vi "Chain3.vi"(7 "Name (\"\" to Use UUID)":string="CSM-Module") -> ()   [LabVIEW 2017, in "CSM-Testcase.lvlib"]
doc: "Creates a template for a CSM module without a user interface.\n\n> [!NOTE] CSM Name Rules\n> - The CSM module name must be unique to avoid entering the \"Critical Error\" state.\n> - If the input is \"\", a UUID will be used as the module name. This module will operate in independent mode and will not be listed in the module list.\n> - If the input ends with '#', the module will run in work mode. Modules with the same name will share the same message queue. External messages will be handled by the idle module.\n\n> [!NOTE] CSM Initialization State\n> - The default value is \"Macro: Initialize\", consistent with the JKISM state machine.\n> - This state is typically not modified and is provided to facilitate external programmatic changes to the initialization state.\n\n\n-- <b>Controls</b> --\n- <b>Name (\"\" to Use UUID)</b>: CSM Module Name\n- <b>Init State(\"Macro: Initialize\")</b>: Initialization State, default is \"Macro: Initialize\""
uses:
  CSM-Testcase.lvlib
  src/user.lib/_NEVSTOP/Communicable State Machine(CSM)/AdvanceAPI/CSM - Revert Arguments-Safe String.vi
  src/user.lib/_NEVSTOP/Communicable State Machine(CSM)/AdvanceAPI/CSM - Make String Arguments Safe.vi
  src/user.lib/_NEVSTOP/Communicable State Machine(CSM)/AdvanceAPI/CSM - Break Down Multiple States String.vi
  src/user.lib/_NEVSTOP/Communicable State Machine(CSM)/AdvanceAPI/CSM - Keywords.vi
  src/user.lib/_NEVSTOP/Communicable State Machine(CSM)/_Shared/Trim Single-line Text.vi
  src/user.lib/_NEVSTOP/Communicable State Machine(CSM)/_Polymophic/Build No-Reply Asynchronous Message with Arguments.vi
  src/user.lib/_NEVSTOP/Communicable State Machine(CSM)/_Polymophic/Build Asynchronous Message with Arguments.vi
  src/user.lib/_NEVSTOP/Communicable State Machine(CSM)/_Polymophic/Build Interrupt Broadcast Message.vi
  src/user.lib/_NEVSTOP/Communicable State Machine(CSM)/_Polymophic/Build Register Message.vi
  src/user.lib/_NEVSTOP/Communicable State Machine(CSM)/Communicable State Machine.lvlib
  src/user.lib/_NEVSTOP/Communicable State Machine(CSM)/addons/Loop-Support/CSM Loop Support.lvlib
panel:
  out "Error Occurred":errorcluster
  out "State History":string
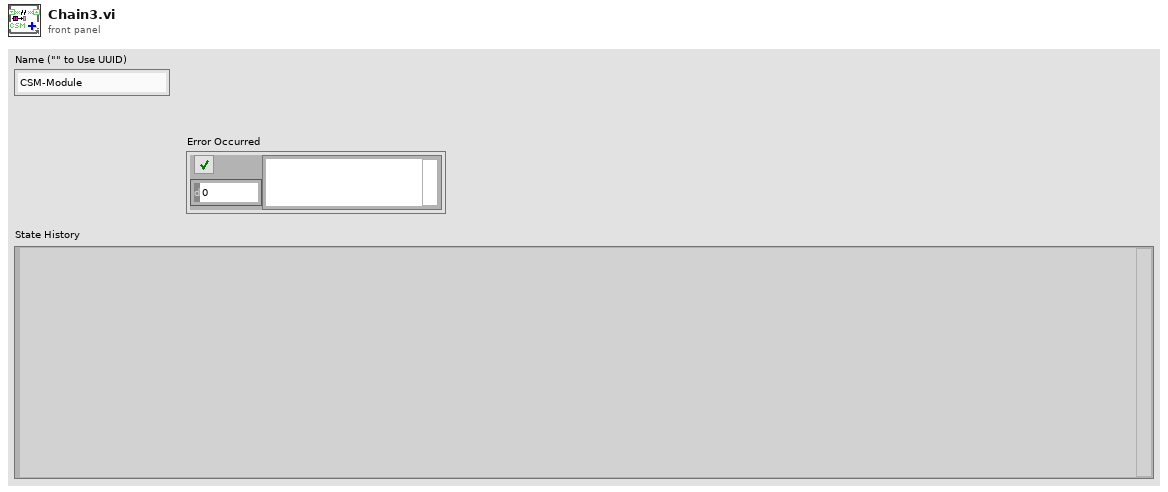
[diagram p1: front panel]
types:
  T1 = cluster{"Arguments":string, "Response":string, "error":errorcluster}
  T2 = enum32{"Invalid", "Standard", "Closed", "Hidden", "Minimized", "Maximized"}
  T3 = enum32{"invalid app kind", "Development System", "Run Time System", "Student Edition", "Embedded LabVIEW", "Evaluation", "Custom"}
  T4 = typedef "Communicable State Machine.lvlib/_CSM_Response Source Message.ctl" = cluster{"‘State":string, "’Arguments":string, "’Error":errorcluster}
  T5 = cluster{"Current VI Reference":refnum<vi>, "Close Panel on Exit?":bool}
  T6 = cluster{"Core":cluster{"Current VI Reference":refnum<vi>, "Close Panel on Exit?":bool}, "Your Boolean data":bool, "Your string data":string, "Counter":u32, "CSM Loop Counter":i32}
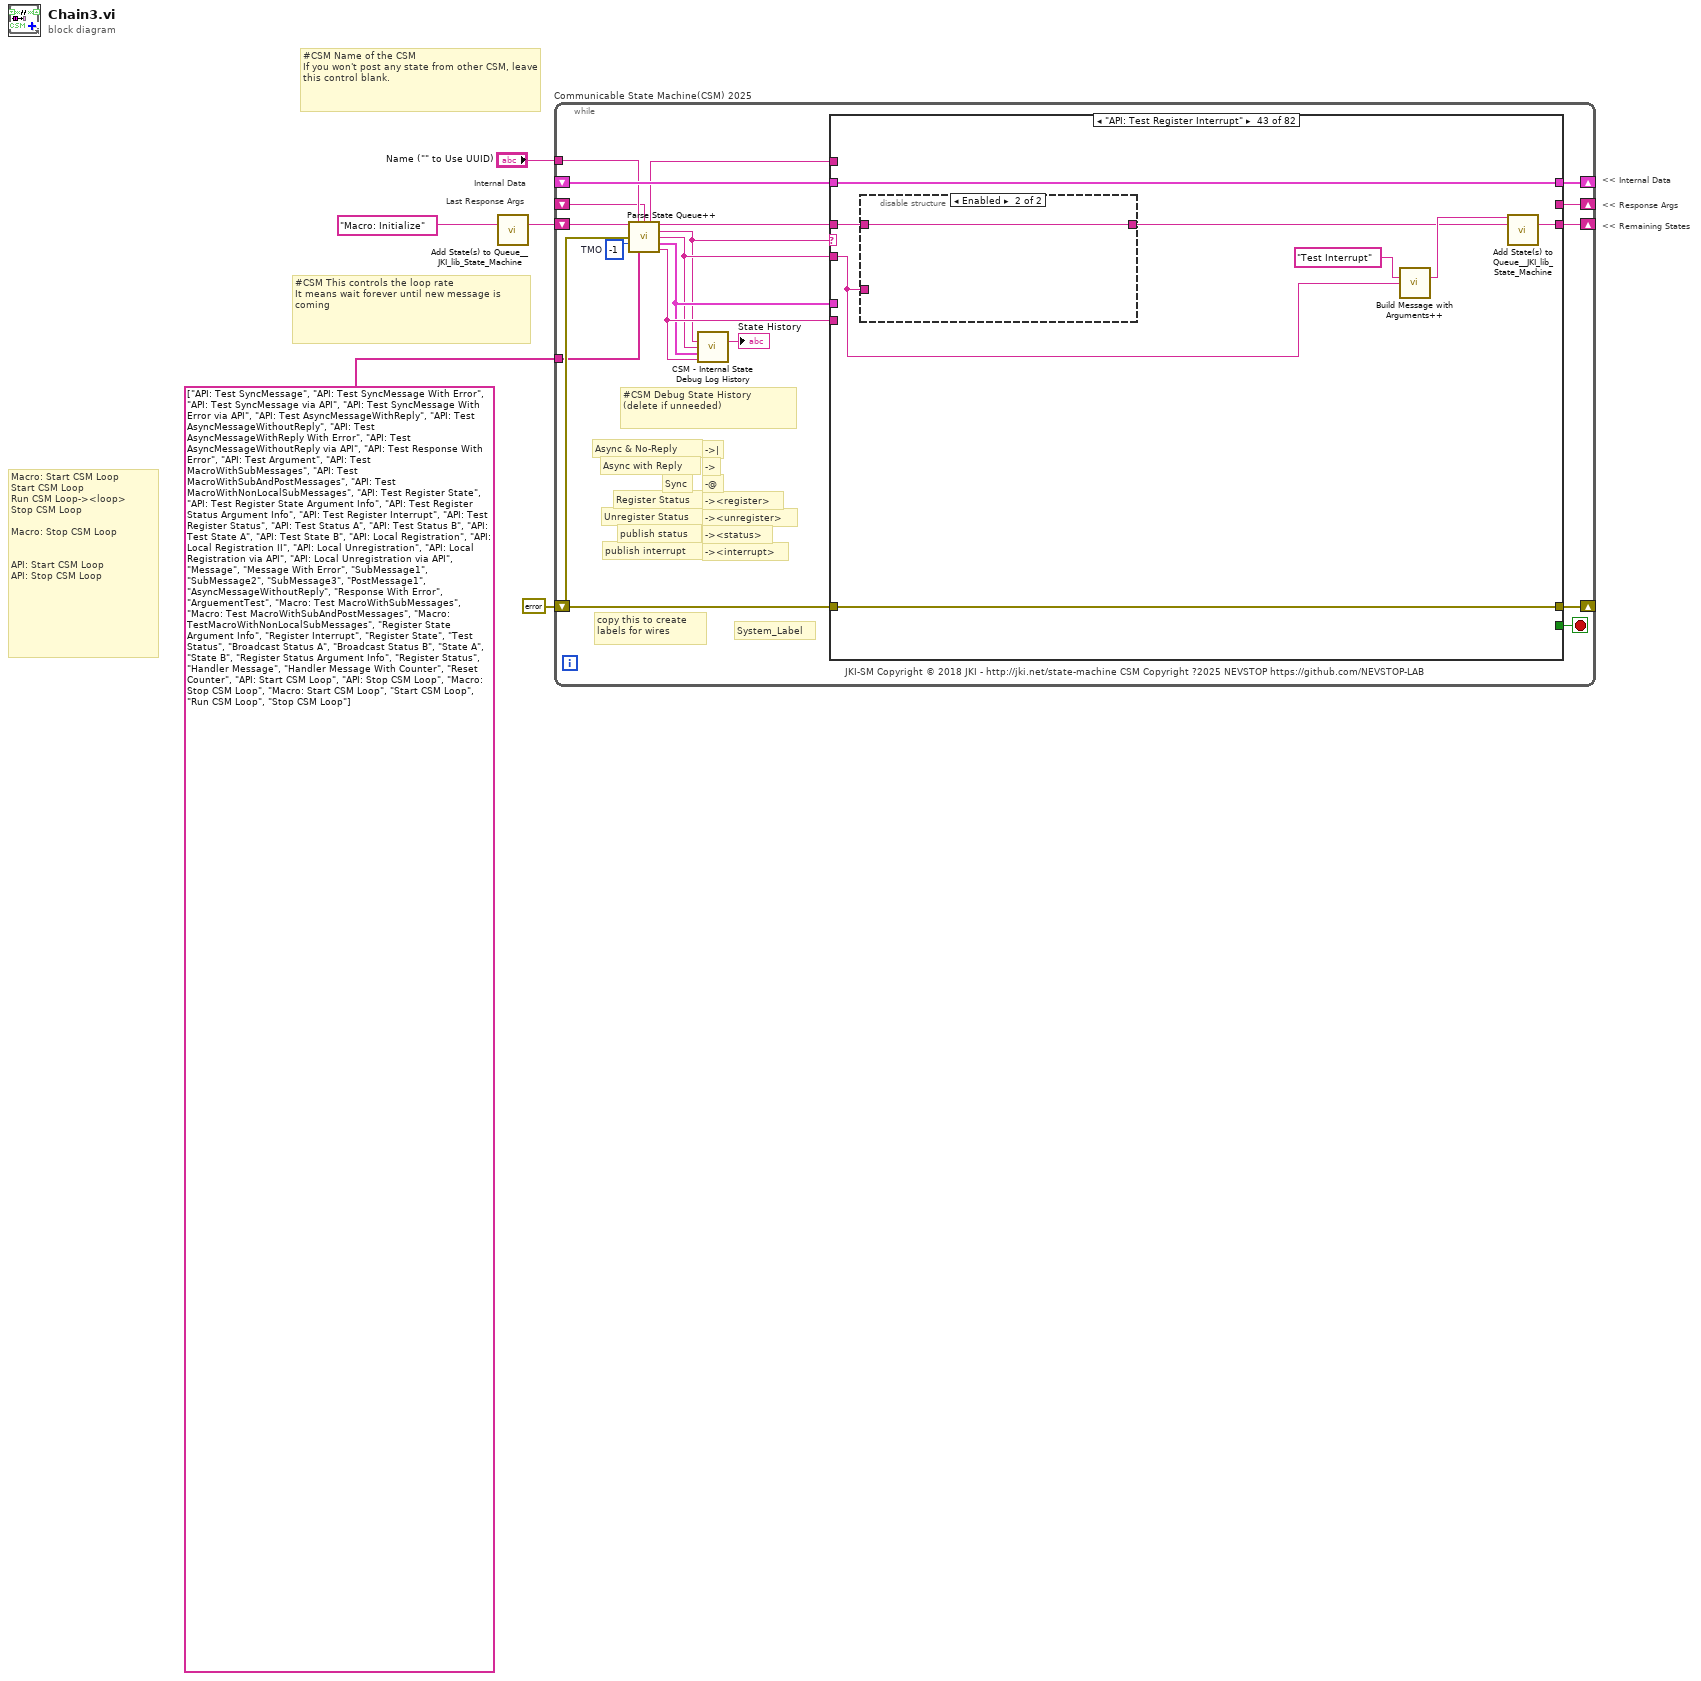
[diagram p0: block diagram]
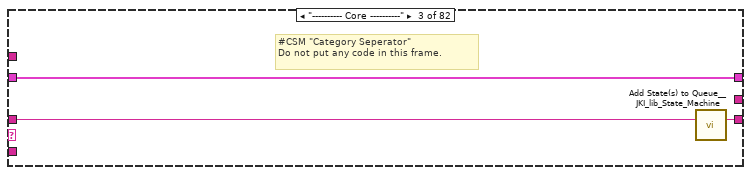
[diagram p4: hidden frame]
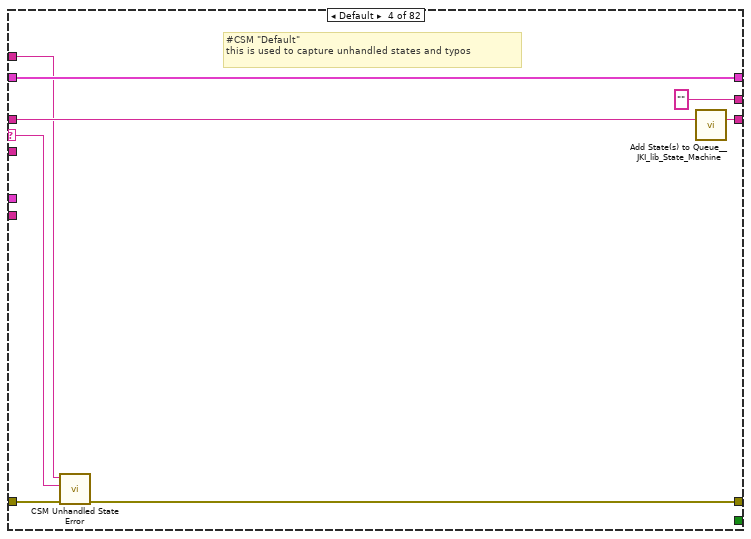
[diagram p5: hidden frame]
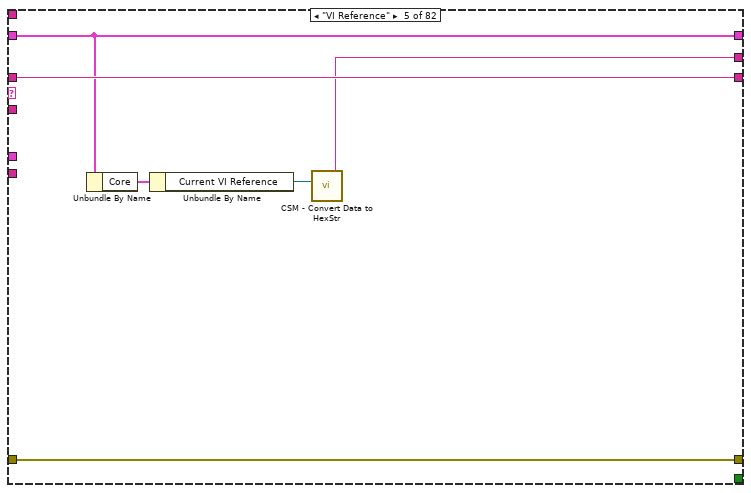
[diagram p6: hidden frame]
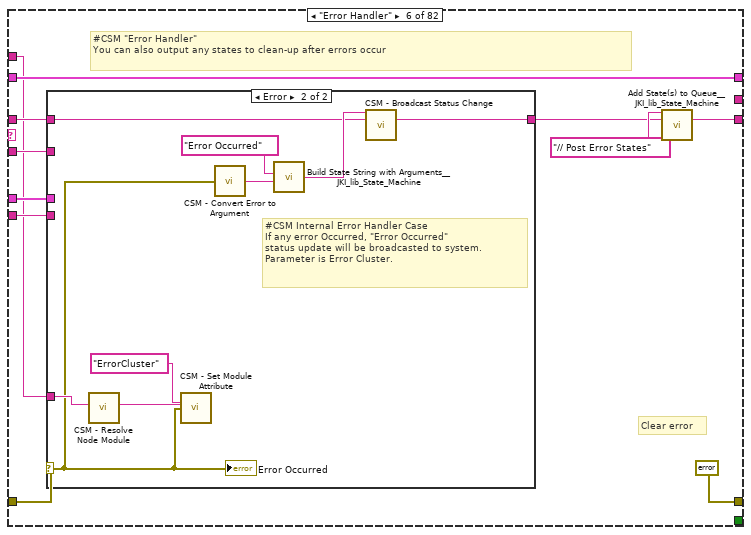
[diagram p7: hidden frame]
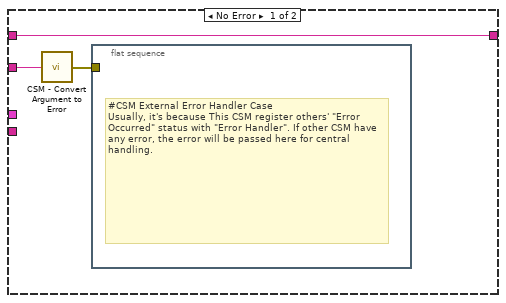
[diagram p8: hidden frame]
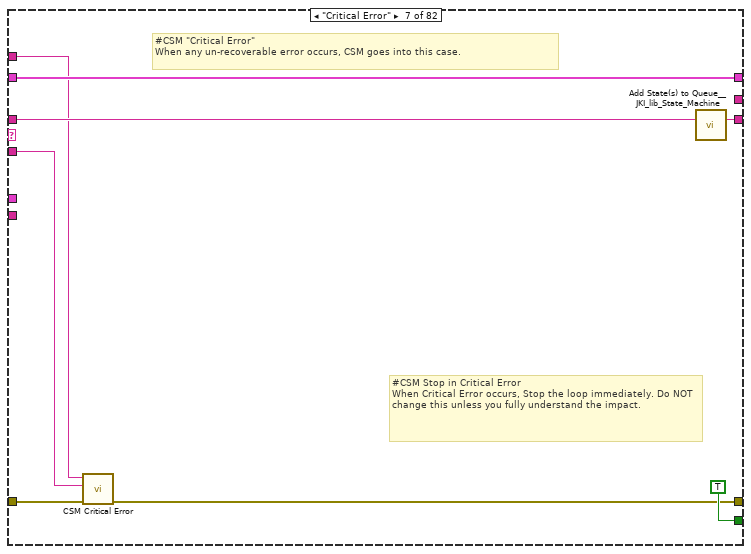
[diagram p9: hidden frame]
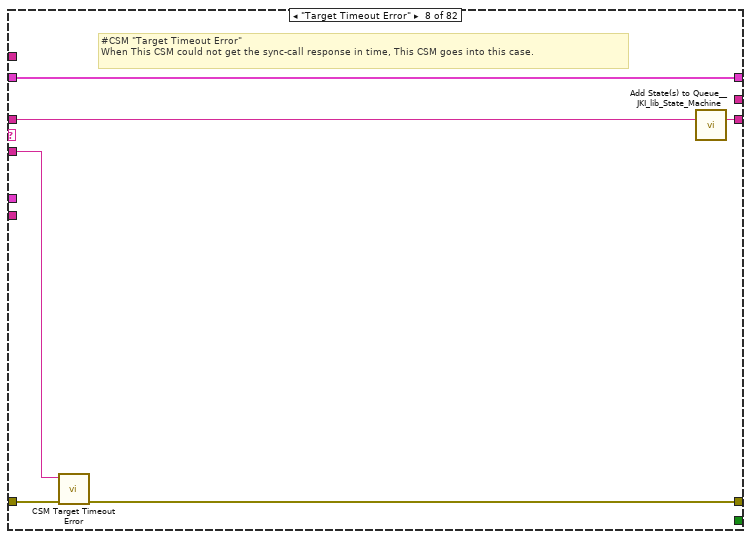
[diagram p10: hidden frame]
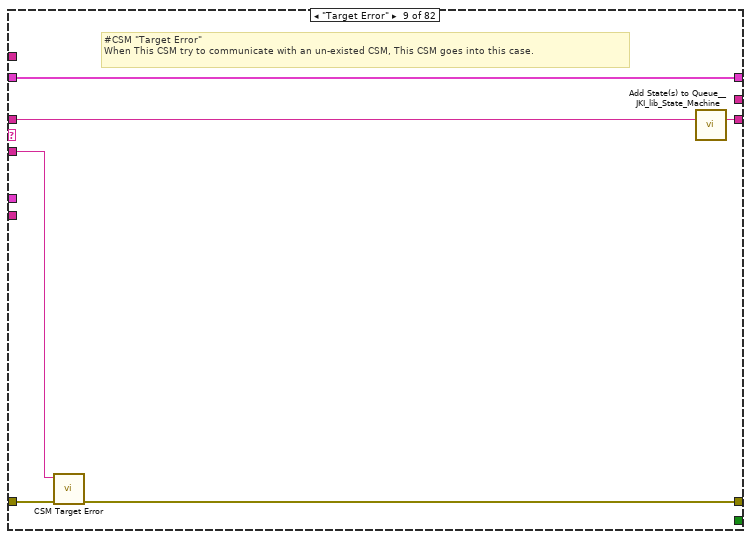
[diagram p11: hidden frame]
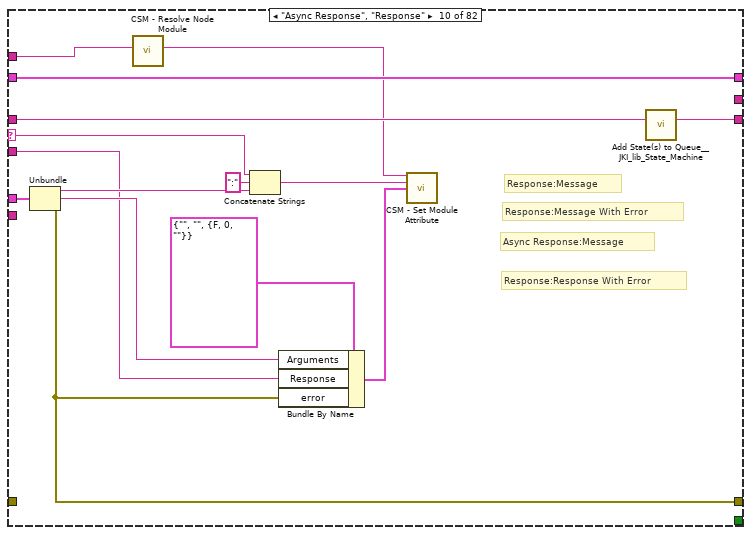
[diagram p12: hidden frame]
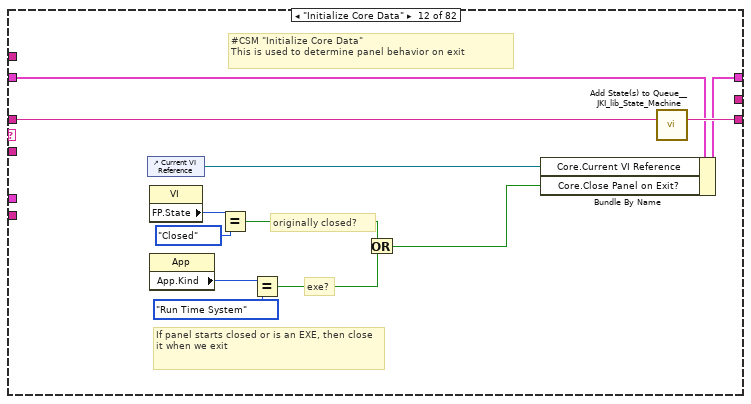
[diagram p14: hidden frame]
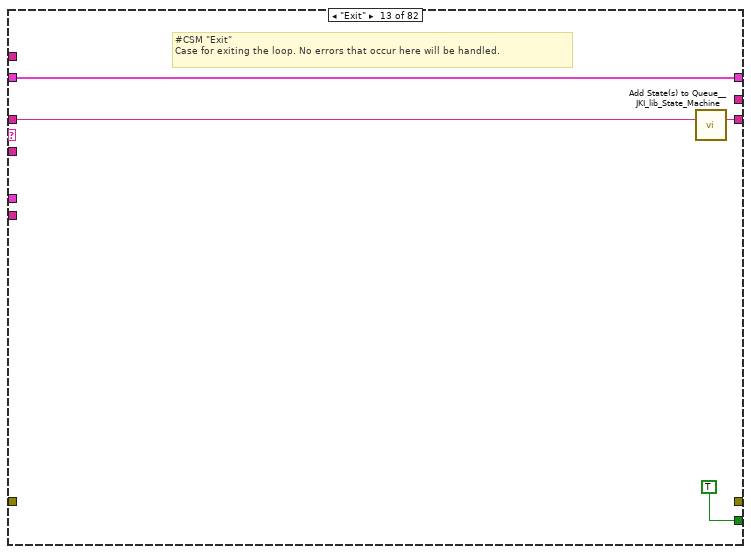
[diagram p15: hidden frame]
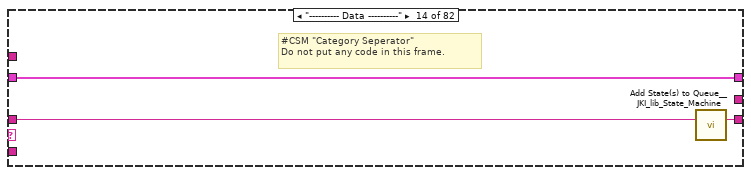
[diagram p16: hidden frame]
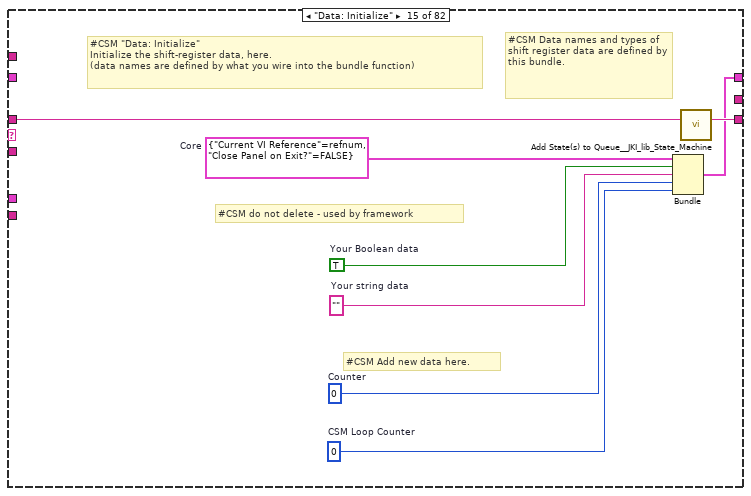
[diagram p17: hidden frame]
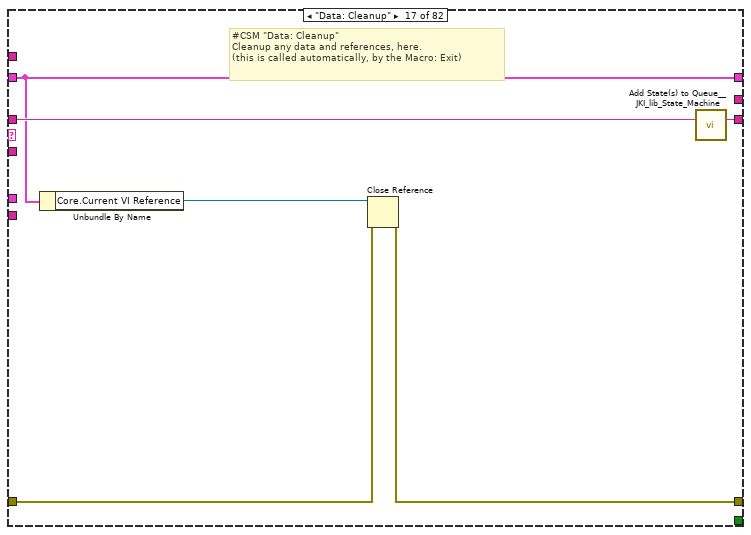
[diagram p19: hidden frame]
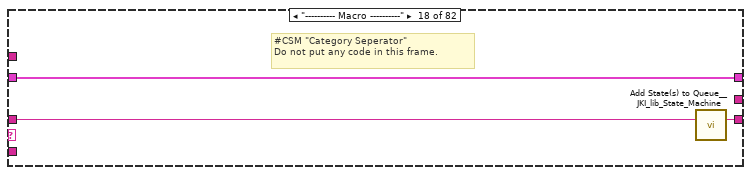
[diagram p20: hidden frame]
diagram:
  # "Macro: Start CSM Loop\nStart CSM Loop\nRun CSM Loop-><loop>\nStop CSM Loop\n\nMacro: Stop CSM Loop\n\n\nAPI: Start CSM Loop\nAPI: Stop CSM Loop"
  # "Last Response Args"
  # "Internal Data"
  # "#CSM Name of the CSM\nIf you won't post any state from other CSM, leave this control blank."
  # "#CSM This controls the loop rate\nIt means wait forever until new message is coming"
  # "<< Internal Data"
  # "<< Response Args"
  # "<< Remaining States"
  n1 = call <vilib>:"Add State(s) to Queue__JKI_lib_State_Machine.vi"("State(s) in (\"\")"="Macro: Initialize" ("Init State(\"Macro: Initialize\")")) -> ("States Out"=w5:string)  [unwired: 14 in]
  n2 = while "Communicable State Machine(CSM) 2025" {
    shift-right: [w19] -> _
    shift-left: _ -> [w18]
    shift-right: [w22] -> _
    shift-left: errorcluster {"status"=FALSE, "code"=0, "source"=""} ("error out") -> [w8]
    shift-right: [w21] -> _
    shift-left: w5 -> [w23]
    tunnel: "Name (\"\" to Use UUID)" -> [w15]
    shift-right: [w16] -> _
    shift-left: _ -> [w10]
    tunnel: string[] ["API: Test SyncMessage", "API: Test SyncMessage With Error", "API: Test SyncMessage via API", "API: Test SyncMessage With Error via API", "API: Test AsyncMessageWithReply", "API: Test AsyncMessageWithoutReply", "API: Test AsyncMessageWithReply With Error", "API: Test AsyncMessageWithoutReply via API", "API: Test Response With Error", "API: Test Argument", "API: Test MacroWithSubMessages", "API: Test MacroWithSubAndPostMessages", "API: Test MacroWithNonLocalSubMessages", "API: Test Register State", "API: Test Register State Argument Info", "API: Test Register Status Argument Info", "API: Test Register Interrupt", "API: Test Register Status", "API: Test Status A", "API: Test Status B", "API: Test State A", "API: Test State B", "API: Local Registration", "API: Local Registration II", "API: Local Unregistration", "API: Local Registration via API", "API: Local Unregistration via API", "Message", "Message With Error", "SubMessage1", "SubMessage2", "SubMessage3", "PostMessage1", "AsyncMessageWithoutReply", "Response With Error", "ArguementTest", "Macro: Test MacroWithSubMessages", "Macro: Test MacroWithSubAndPostMessages", "Macro: TestMacroWithNonLocalSubMessages", "Register State Argument Info", "Register Interrupt", "Register State", "Test Status", "Broadcast Status A", "Broadcast Status B", "State A", "State B", "Register Status Argument Info", "Register Status", "Handler Message", "Handler Message With Counter", "Reset Counter", "API: Start CSM Loop", "API: Stop CSM Loop", "Macro: Stop CSM Loop", "Macro: Start CSM Loop", "Start CSM Loop", "Run CSM Loop", "Stop CSM Loop"] ("Allowed Messages (Empty for All)") -> [w6]
    stop <- w20 stop-if-true
    w17 = -1  # TMO
    # "#CSM Debug State History\n(delete if unneeded)"
    # "-><interrupt>"
    # "-><status>"
    # "-><unregister>"
    # "-><register>"
    # "-@"
    # "->"
    # "->|"
    # "publish interrupt"
    # "publish status"
    # "Unregister Status"
    # "Register Status"
    # "Sync"
    # "Async with Reply"
    # "Async & No-Reply"
    # "JKI-SM Copyright © 2018 JKI - http://jki.net/state-machine CSM Copyright ?2025 NEVSTOP https://github.com/NEVSTOP-LAB"
    # "copy this to create labels for wires"
    # "System_Label"
    n3 = call "Parse State Queue++.vi"("State Queue"=w23, "Name (\"\" to Use UUID)"=w15, "Response Arguments"=w10, "Previous Error"=w8, "Dequeue (1 ms)"=w17, "Allowed Messages (Empty for All)"=w6) -> ("Name Used"=w9:string, "Remaining States"=w24:string, "Current State"=w11:string, "Arguments"=w12:string, "Additional Information"=w13:T4, "Source CSM"=w14:string)  [unwired: 4 in]
    n4 = call "CSM - Internal State Debug Log History.vi"("State"=w11, "Arguments (\"\")"=w12, ">> Response Source Message >>"=w13, "Source (\"\")"=w14) -> ("Debug Log"=→"State History":string)  [unwired: 11 in]
    n5 = case shown="\"API: Test Register Interrupt\"" w11 {
      selector: w11 -> [_ _ _ w35 _ _ _ _ _ w99 _ _ _ _ _ _ _ _ _ _ _ _ _ _ _ _ _ _ _ _ _ _ _ _ _ _ _ _ _ _ _ _ _ _ _ _ _ _ _ _ _ _ _ _ _ _ _ _ _ w565 w575 _ w589 _ _ _ _ _ _ _ _ _ _ w655 _ _ _ w679 w690 w697 w712 _]
      tunnel: w24 -> [w25 w28 w31 w39 w44 w50 w76 w82 w88 w103 w105 w117 w121 w124 w132 w134 w140 w143 w147 w153 w157 w162 w176 w196 w225 w229 w233 w245 w270 w298 w313 w325 w337 w351 w374 w385 w398 w405 w412 w419 w426 w431 w445 w461 w468 w475 w482 w489 w500 w508 w517 w526 w535 w538 w542 w549 w554 w557 w561 w573 w583 w588 w594 w601 w604 w616 w622 w628 w632 w637 w641 w645 w649 w658 w662 w670 w676 w683 w692 w701 w716 w726]
      tunnel: w12 -> [_ _ _ _ _ w49 w72 w79 w85 w93 _ _ _ _ _ _ _ _ _ _ _ _ w163 w183 w208 _ w236 w248 w273 w301 w316 w328 w340 w354 w370 w388 w395 w402 w409 w416 w423 w430 w444 w458 w465 w472 w479 w486 w493 _ w510 w518 w527 _ _ w547 _ _ _ _ _ w585 _ w597 w606 _ w618 w624 w630 w635 w640 w644 w648 w654 w661 w668 w674 w680 w691 w696 w707 _]
      tunnel: w18 -> [w26 w27 w29 w37 w43 w55 w74 w80 w86 w101 w104 w111 w119 w122 _ w133 w135 w141 w145 w151 w158 w160 w178 w198 w227 w228 w237 w249 w274 w302 w317 w329 w341 w355 w377 w389 w400 w407 w414 w421 w428 w436 w450 w463 w470 w477 w484 w491 w498 w506 w515 w524 w533 w539 w544 w548 w552 w555 w560 w571 w581 w586 w595 w602 w608 w617 w623 w629 w634 w639 w642 w646 w650 w659 w663 w669 w675 w684 w693 w702 w709 w724]
      tunnel: [_ _ _ w32 w45 errorcluster {"status"=FALSE, "code"=0, "source"=""} ("error out") w69 w77 w83 w92 _ _ _ _ _ _ w136 _ _ _ _ _ _ _ _ _ w230 w242 w267 w295 w310 w322 w334 w347 w371 w382 w399 w406 w413 w420 w427 w435 w449 w462 w469 w476 w483 w490 _ _ _ w522 w531 w540 w545 _ _ _ w562 w563 w578 _ _ _ _ _ _ _ w633 w638 w643 w647 w651 w653 w664 w665 w671 w678 w687 w698 w713 _] -> w22
      tunnel: w8 -> [_ _ _ w33 w45 w53 w70 w78 w84 _ _ _ _ _ _ _ w137 _ _ _ _ _ _ _ _ _ _ _ _ _ _ _ _ _ _ _ w399 w406 w413 w420 w427 w435 w449 w462 w469 w476 w483 w490 _ _ _ _ _ w540 w545 _ _ _ w562 _ _ _ _ _ _ _ _ _ w633 w638 w643 w647 w651 w660 w664 w666 w672 w685 w694 w703 w717 _]
      tunnel: [w25 w28 w30 w38 w44 w51 w75 w81 w87 w102 w105 w116 w120 w123 w131 w134 w139 w142 w146 w152 w154 w161 w177 w197 w226 w229 w234 w246 w271 w299 w314 w326 w338 w352 w375 w386 w397 w404 w411 w418 w425 w429 w443 w460 w467 w474 w481 w488 w499 w507 w516 w525 w534 w537 w541 w549 w553 w556 w561 w574 w584 w587 w596 w598 w603 w614 w619 w625 w631 w636 w641 w645 w649 w658 w662 w670 w676 w683 w692 w701 w716 w725] -> w21
      tunnel: [_ _ _ _ _ _ TRUE _ _ _ _ _ TRUE _ _ _ _ _ _ _ _ _ _ _ _ _ _ _ _ _ _ _ _ _ _ _ _ _ _ _ _ _ _ _ _ _ _ _ _ _ _ _ _ _ _ _ _ _ _ _ _ _ _ _ _ _ _ _ _ _ _ _ _ _ _ _ _ _ _ _ _ _] -> w20
      tunnel: [w26 w27 w29 w37 w43 w55 w74 w80 w86 w101 w104 w115 w119 w122 w130 w133 w135 w141 w145 w151 w158 w160 w178 w198 w227 w228 w237 w249 w274 w302 w317 w329 w341 w355 w377 w389 w400 w407 w414 w421 w428 w436 w450 w463 w470 w477 w484 w491 w498 w506 w515 w524 w533 w539 w544 w548 w552 w555 w559 w569 w580 w586 w595 w602 w608 w617 w623 w629 w634 w639 w642 w646 w650 w659 w663 w669 w675 w684 w693 w702 w708 w722] -> w19
      tunnel: w14 -> [_ _ _ _ _ w48 _ _ _ _ _ _ _ _ _ _ _ _ _ _ _ _ _ _ _ _ _ _ _ _ _ _ _ _ _ _ _ _ _ _ _ _ _ _ _ _ _ _ _ _ _ _ _ _ _ _ _ _ _ _ _ _ _ _ _ _ _ _ _ _ _ _ _ _ _ _ _ _ _ _ _ _]
      tunnel: w13 -> [_ _ _ _ _ w47 _ _ _ w100 _ _ _ _ _ _ _ _ _ _ _ _ _ _ _ _ _ _ _ _ _ _ _ _ _ _ _ _ _ _ _ _ _ _ _ _ _ _ _ _ _ _ _ _ _ _ _ _ _ _ _ _ _ _ _ _ _ _ _ _ _ _ _ _ _ _ _ _ _ _ _ _]
      tunnel: [_ _ _ "" w40 _ _ _ _ _ _ _ _ _ _ _ _ _ _ _ _ _ _ _ _ _ _ _ _ _ _ _ _ _ _ _ _ _ _ _ _ _ _ _ _ _ _ _ _ _ _ _ _ _ _ w546 _ _ _ _ _ w585 w590 _ _ _ _ _ w630 w635 w640 w644 w648 w654 w661 w668 w674 _ w691 w696 _ _] -> w16
      tunnel: w9 -> [_ _ _ w34 _ w46 w71 _ _ w90 _ _ _ _ _ _ _ _ _ _ _ _ _ _ _ _ _ _ w258 w286 _ _ _ w348 _ _ _ _ _ _ _ _ _ _ _ _ _ _ w496 w504 w513 w523 w532 _ _ _ _ _ _ w567 w577 _ w591 _ _ w611 _ _ _ _ _ _ _ w657 _ _ _ w682 w689 w700 w715 _]
      frame "", "Idle" {
        # "#CSM \"Idle/Event Handler\"\nexecutes when the state queue is empty"
      }
      frame "CSM Documentation" {
        # "#CSM State Syntax\n\n// Comment line, all text to the right of “//” will be ignored\n// Local Message Example\nDoSth: DoA >> Arguments\n\n// Sync Call Example\nAPI: xxxx >> Arguments -@ TargetModule\n\n// Async Call Example\nAPI: xxxx >> Arguments -> TargetModule\n\n// Async Call without Reply Example\nAPI: xxxx >> Arguments ->| TargetModule\n\n// Broadcast normal status:\nStatus >> StatusArguments  -><status>\n\n// Broadcast Interrupt status:\nInterrupt >> StatusArguments  -><interrupt>\n\n// Register Source Module's status to Handler Module\nStatus@Source Module >> Handler Module@Handler Module -><register>\n\n// Unegister Source Module's status\nStatus@Source Module >> Handler Module -><unregister>"
        # "#CSM README FIRST\n\nCommunicable State Machine(CSM) is a LabVIEW application framework that builds upon JKI State Machine(JKISM). It follows the pattern of JKISM and extends the keywords to describe message communication between modules, including concepts such as Sync-Message, Async-Message, Subscription/Unsubscription of status - essential elements for creating reusable code modules. For more information, please visit the CSM wiki: https://nevstop-lab.github.io/CSM-Wiki/\n\nFor instructions on JKI State Machine, visit: \n    http://jki.net/state-machine/\nFor information about CSM, visit: \n    https://github.com/NEVSTOP-LAB"
        # "#CSM \"Documentation\"\nCase for holding CSM Documenation"
      }
      frame "---------- Core ----------" {
        # "#CSM \"Category Seperator\"\nDo not put any code in this frame."
        n6 = call <vilib>:"Add State(s) to Queue__JKI_lib_State_Machine.vi"("State(s) in (\"\")"=w31) -> ("States Out"=w30:string)  [unwired: 14 in]
      }
      frame Default {
        # "#CSM \"Default\"\nthis is used to capture unhandled states and typos"
        n7 = call "CSM Unhandled State Error.vi"("error in (no error)"=w33, "Undefined State"=w35, "CSM Name"=w34) -> ("error out"=w32:errorcluster)  [unwired: 8 in]
        n8 = call <vilib>:"Add State(s) to Queue__JKI_lib_State_Machine.vi"("State(s) in (\"\")"=w39) -> ("States Out"=w38:string)  [unwired: 14 in]
      }
      frame "VI Reference" {
        n9 = Unbundle By Name(w43) -> ("Core"=w42:T5)
        n10 = Unbundle By Name(w42) -> ("Current VI Reference"=w41:refnum<vi>)
        n11 = call "CSM - Convert Data to HexStr.vi"("Variant"=w41) -> ("HEX String (0-9,A-F)"=w40:string)  [unwired: 8 in]
      }
      frame "Error Handler" {
        # "#CSM \"Error Handler\"\nYou can also output any states to clean-up after errors occur"
        # "Clear error"
        n12 = case shown="Error" w53 {
          selector: w53 -> [_ w61]
          tunnel: [w59 w65] -> w52
          tunnel: w50 -> [w59 w64]
          tunnel: w49 -> [w58 _]
          tunnel: w48 -> [_ _]
          tunnel: w47 -> [_ _]
          tunnel: w46 -> [_ w63]
          frame No Error {
            n13 = call "CSM - Convert Argument to Error.vi"("Argument"=w58) -> ("Error"=w57:errorcluster)  [unwired: 4 in]
            n14 = flat-sequence {
              tunnel: w57 -> [_]
              frame #0 {
                # "#CSM External Error Handler Case\nUsually, it's because This CSM register others' \"Error Occurred\" status with \"Error Handler\". If other CSM have any error, the error will be passed here for central handling."
              }
            }
          }
          frame Error {
            # "#CSM Internal Error Handler Case \nIf any error Occurred, \"Error Occurred\" \nstatus update will be broadcasted to system.\nParameter is Error Cluster."
            n15 = call "CSM - Resolve Node Module.vi"("Node Name"=w63) -> ("CSM Module Name"=w62:string)  [unwired: 10 in]
            n16 = call "CSM - Set Module Attribute.vi"("CSM Name"=w62, "Attribute"="ErrorCluster", "Value"=w61) -> ()  [unwired: 9 in, 4 out]
            n17 = call "CSM - Convert Error to Argument.vi"("Error"=w61) -> ("Argument"=w67:string)  [unwired: 4 in]
            n18 = call <vilib>:"Build State String with Arguments__JKI_lib_State_Machine.vi"("Arguments (\"\")"=w67, "State"="Error Occurred" ("Status with Arguments")) -> ("State with Arguments"=w66:string)  [unwired: 4 in]
            n19 = call "CSM - Broadcast Status Change.vi"("Status With Arguments"=w66, "State Queue"=w64) -> ("Remaining States"=w65:string)  [unwired: 13 in]
            "Error Occurred" <- w61
          }
        }
        n20 = call <vilib>:"Add State(s) to Queue__JKI_lib_State_Machine.vi"("State(s) in Front (\"\")"="// Post Error States", "State(s) in (\"\")"=w52) -> ("States Out"=w51:string)  [unwired: 13 in]
      }
      frame "Critical Error" {
        # "#CSM \"Critical Error\"\nWhen any un-recoverable error occurs, CSM goes into this case."
        # "#CSM Stop in Critical Error\nWhen Critical Error occurs, Stop the loop immediately. Do NOT change this unless you fully understand the impact."
        n21 = call "CSM Critical Error.vi"("error in (no error)"=w70, "Arugments (As Reason)"=w72, "CSM Name"=w71) -> ("error out"=w69:errorcluster)  [unwired: 8 in]
        n22 = call <vilib>:"Add State(s) to Queue__JKI_lib_State_Machine.vi"("State(s) in (\"\")"=w76) -> ("States Out"=w75:string)  [unwired: 14 in]
      }
      frame "Target Timeout Error" {
        # "#CSM \"Target Timeout Error\"\nWhen This CSM could not get the sync-call response in time, This CSM goes into this case."
        n23 = call "CSM Target Timeout Error.vi"("error in (no error)"=w78, "Arguments (As CSM Name)"=w79) -> ("error out"=w77:errorcluster)  [unwired: 9 in]
        n24 = call <vilib>:"Add State(s) to Queue__JKI_lib_State_Machine.vi"("State(s) in (\"\")"=w82) -> ("States Out"=w81:string)  [unwired: 14 in]
      }
      frame "Target Error" {
        # "#CSM \"Target Error\"\nWhen This CSM try to communicate with an un-existed CSM, This CSM goes into this case."
        n25 = call "CSM Target Error.vi"("error in (no error)"=w84, "Arguments (As CSM Name)"=w85) -> ("error out"=w83:errorcluster)  [unwired: 9 in]
        n26 = call <vilib>:"Add State(s) to Queue__JKI_lib_State_Machine.vi"("State(s) in (\"\")"=w88) -> ("States Out"=w87:string)  [unwired: 14 in]
      }
      frame "Async Response", "Response" {
        # "Response:Response With Error"
        # "Response:Message With Error"
        # "Async Response:Message"
        # "Response:Message"
        n27 = Unbundle(w100) -> ("‘State"=w98:string, "’Arguments"=w94:string, "’Error"=w92:errorcluster)
        n28 = call "CSM - Resolve Node Module.vi"("Node Name"=w90) -> ("CSM Module Name"=w89:string)  [unwired: 10 in]
        n29 = Concatenate Strings(w99, ":" ("string"), w98) -> (w96:string)
        n30 = Bundle By Name(cluster=T1 {"Arguments"="", "Response"="", "error"={"status"=FALSE, "code"=0, "source"=""}}, "Arguments"=w94, "Response"=w93, "error"=w92) -> (w91:T1)
        n31 = call "CSM - Set Module Attribute.vi"("CSM Name"=w89, "Attribute"=w96, "Value"=w91) -> ()  [unwired: 9 in, 4 out]
        n32 = call <vilib>:"Add State(s) to Queue__JKI_lib_State_Machine.vi"("State(s) in (\"\")"=w103) -> ("States Out"=w102:string)  [unwired: 14 in]
      }
      frame "Async Message Posted" {
        # "#CSM \"Async Message Posted\"\nAfter Async Message is posted (-> or ->| ), CSM goes to this state for post-action.\nYou can use Argument - State to tell which Async Message is called."
      }
      frame "Initialize Core Data" {
        # "#CSM \"Initialize Core Data\"\nThis is used to determine panel behavior on exit"
        # "originally closed?"
        # "exe?"
        # "If panel starts closed or is an EXE, then close it when we exit"
        n33 = control-ref of="Current VI Reference"() -> (w109:refnum<vi>)
        n34 = property class="VI"() -> ("FP.State"=w108:T2)  [unwired: 2 in, 2 out]
        n35 = property class="App"() -> ("App.Kind"=w114:T3)  [unwired: 2 in, 2 out]
        n36 = Equal?(x=w108, y=T2."Closed" ("Front Panel Window:State")) -> (x = y?=w106:bool)
        n37 = Equal?(x=w114, y=T3."Run Time System" ("Application:Kind")) -> (x = y?=w112:bool)
        n38 = Or(x=w106, y=w112) -> (x .or. y?=w110:bool)
        n39 = Bundle By Name(cluster=w111, "Core.Current VI Reference"=w109, "Core.Close Panel on Exit?"=w110) -> (w115:T6)
        n40 = call <vilib>:"Add State(s) to Queue__JKI_lib_State_Machine.vi"("State(s) in (\"\")"=w117) -> ("States Out"=w116:string)  [unwired: 14 in]
      }
      frame "Exit" {
        # "#CSM \"Exit\"\nCase for exiting the loop. No errors that occur here will be handled."
        n41 = call <vilib>:"Add State(s) to Queue__JKI_lib_State_Machine.vi"("State(s) in (\"\")"=w121) -> ("States Out"=w120:string)  [unwired: 14 in]
      }
      frame "---------- Data ----------" {
        # "#CSM \"Category Seperator\"\nDo not put any code in this frame."
        n42 = call <vilib>:"Add State(s) to Queue__JKI_lib_State_Machine.vi"("State(s) in (\"\")"=w124) -> ("States Out"=w123:string)  [unwired: 14 in]
      }
      frame "Data: Initialize" {
        w125 = 0  # CSM Loop Counter
        w126 = u32 0  # Counter
        w127 = T5 {"Current VI Reference"=refnum, "Close Panel on Exit?"=FALSE}  # Core
        w129 = TRUE  # Your Boolean data
        w128 = ""  # Your string data
        # "#CSM \"Data: Initialize\"\nInitialize the shift-register data, here.\n(data names are defined by what you wire into the bundle function)"
        # "#CSM do not delete - used by framework"
        # "#CSM Add new data here."
        # "#CSM Data names and types of shift register data are defined by this bundle."
        n43 = Bundle("Core"=w127, "Your Boolean data"=w129, "Your string data"=w128, "Counter"=w126, "CSM Loop Counter"=w125) -> (w130:T6)  [unwired: 1 in]
        n44 = call <vilib>:"Add State(s) to Queue__JKI_lib_State_Machine.vi"("State(s) in (\"\")"=w132) -> ("States Out"=w131:string)  [unwired: 14 in]
      }
      frame "Data: Update Indicators" {
      }
      frame "Data: Cleanup" {
        # "#CSM \"Data: Cleanup\"\nCleanup any data and references, here.\n(this is called automatically, by the Macro: Exit)"
        n45 = Unbundle By Name(w135) -> ("Core.Current VI Reference"=w138:refnum<vi>)
        n46 = Close Reference(reference=w138, error in (no error)=w137) -> (error out=w136:errorcluster)
        n47 = call <vilib>:"Add State(s) to Queue__JKI_lib_State_Machine.vi"("State(s) in (\"\")"=w140) -> ("States Out"=w139:string)  [unwired: 14 in]
      }
      frame "---------- Macro ----------" {
        # "#CSM \"Category Seperator\"\nDo not put any code in this frame."
        n48 = call <vilib>:"Add State(s) to Queue__JKI_lib_State_Machine.vi"("State(s) in (\"\")"=w143) -> ("States Out"=w142:string)  [unwired: 14 in]
      }
      frame "Macro: Initialize" {
        # "#CSM \"Macro: Initialize\"\nInitialization Macro (This is called once, when the VI starts)"
        n49 = call <vilib>:"Add State(s) to Queue__JKI_lib_State_Machine.vi"("State(s) in Front (\"\")"="Data: Initialize\nInitialize Core Data\nData: Update Indicators", "State(s) in (\"\")"=w147) -> ("States Out"=w146:string)  [unwired: 13 in]
      }
      frame "Macro: Exit" {
        # "#CSM \"Macro: Exit\"\nExit Macro (This is called once, when the VI exits)"
        n50 = call <vilib>:"Add State(s) to Queue__JKI_lib_State_Machine.vi"("State(s) in Front (\"\")"="//Exit Sub-Modules ", "State(s) at Back (\"\")"="Data: Cleanup\nExit") -> ("States Out"=w149:string)  [unwired: 13 in]
        n51 = call <vilib>:"Add State(s) to Queue__JKI_lib_State_Machine.vi"("State(s) in Front (\"\")"=w149, "State(s) in (\"\")"=w153) -> ("States Out"=w152:string)  [unwired: 13 in]
      }
      frame "Macro: Start CSM Loop" {
        n52 = call "CSMLS - Define Loop State(s).vi"("Loop States"="Start CSM Loop\nRun CSM Loop-><loop>\nStop CSM Loop", "States Queue"=w157, "Add to Front? (F)"=FALSE) -> ("Remaining States"=w154:string)  [unwired: 12 in]
      }
      frame "Macro: Stop CSM Loop" {
        n53 = call <vilib>:"Add State(s) to Queue__JKI_lib_State_Machine.vi"("State(s) in Front (\"\")"="Stop CSM Loop", "State(s) in (\"\")"=w162) -> ("States Out"=w161:string)  [unwired: 13 in]
      }
      frame "Macro: Test MacroWithSubMessages" {
        w164 = "SubMessage2" ("State With Arguments")
        w166 = "SubMessage1" ("State With Arguments")
        n54 = call "uuid.vi"() -> ("UUID"=w165:string)  [unwired: 11 in]
        n55 = call "uuid.vi"() -> ("UUID"=w167:string)  [unwired: 11 in]
        n56 = Concatenate Strings(w166, w167) -> (w168:string)
        n57 = Concatenate Strings(w164, w165) -> (w169:string)
        n58 = call <vilib>:"Build State String with Arguments__JKI_lib_State_Machine.vi"("Arguments (\"\")"=w163, "State"="SubMessage3" ("State With Arguments")) -> ("State with Arguments"=w171:string)  [unwired: 4 in]
        n59 = call <vilib>:"Build State String with Arguments__JKI_lib_State_Machine.vi"("Arguments (\"\")"=w168, "State"=w166) -> ("State with Arguments"=w173:string)  [unwired: 4 in]
        n60 = call <vilib>:"Build State String with Arguments__JKI_lib_State_Machine.vi"("Arguments (\"\")"=w169, "State"=w164) -> ("State with Arguments"=w172:string)  [unwired: 4 in]
        n61 = Build Array(w173, w172, w171) -> (w170:string[])
        n62 = call "CSM - Compact Multiple States.vi"("Multiple States"=w170) -> ("States"=w175:string)  [unwired: 9 in]
        n63 = call <vilib>:"Add State(s) to Queue__JKI_lib_State_Machine.vi"("State(s) in Front (\"\")"=w175, "State(s) in (\"\")"=w176) -> ("States Out"=w177:string)  [unwired: 13 in]
      }
      frame "Macro: Test MacroWithSubAndPostMessages" {
        w182 = "PostMessage1" ("State With Arguments")
        w184 = "SubMessage2" ("State With Arguments")
        w186 = "SubMessage1" ("State With Arguments")
        n64 = call "uuid.vi"() -> ("UUID"=w185:string)  [unwired: 11 in]
        n65 = call "uuid.vi"() -> ("UUID"=w181:string)  [unwired: 11 in]
        n66 = call "uuid.vi"() -> ("UUID"=w187:string)  [unwired: 11 in]
        n67 = Concatenate Strings(w182, w181) -> (w180:string)
        n68 = Concatenate Strings(w186, w187) -> (w188:string)
        n69 = Concatenate Strings(w184, w185) -> (w189:string)
        n70 = call <vilib>:"Build State String with Arguments__JKI_lib_State_Machine.vi"("Arguments (\"\")"=w183, "State"="SubMessage3" ("State With Arguments")) -> ("State with Arguments"=w191:string)  [unwired: 4 in]
        n71 = call <vilib>:"Build State String with Arguments__JKI_lib_State_Machine.vi"("Arguments (\"\")"=w180, "State"=w182) -> ("State with Arguments"=w179:string)  [unwired: 4 in]
        n72 = call <vilib>:"Build State String with Arguments__JKI_lib_State_Machine.vi"("Arguments (\"\")"=w188, "State"=w186) -> ("State with Arguments"=w193:string)  [unwired: 4 in]
        n73 = call <vilib>:"Build State String with Arguments__JKI_lib_State_Machine.vi"("Arguments (\"\")"=w189, "State"=w184) -> ("State with Arguments"=w192:string)  [unwired: 4 in]
        n74 = Build Array(w193, w192, w191) -> (w190:string[])
        n75 = call "CSM - Compact Multiple States.vi"("Multiple States"=w190) -> ("States"=w195:string)  [unwired: 9 in]
        n76 = call <vilib>:"Add State(s) to Queue__JKI_lib_State_Machine.vi"("State(s) in Front (\"\")"=w195, "State(s) in (\"\")"=w196, "State(s) at Back (\"\")"=w179) -> ("States Out"=w197:string)  [unwired: 12 in]
      }
      frame "Macro: TestMacroWithNonLocalSubMessages" {
        w212 = "PostMessage1" ("State With Arguments")
        w213 = "SubMessage2" ("State With Arguments")
        w215 = "SubMessage1" ("State With Arguments")
        n77 = Match Pattern(string=w208, regular expression="+") -> (before substring=w200:string, after substring=w199:string)  [unwired: 1 in, 2 out]
        n78 = call "uuid.vi"() -> ("UUID"=w211:string)  [unwired: 11 in]
        n79 = call "uuid.vi"() -> ("UUID"=w214:string)  [unwired: 11 in]
        n80 = call "uuid.vi"() -> ("UUID"=w216:string)  [unwired: 11 in]
        n81 = Concatenate Strings(w212, w211) -> (w210:string)
        n82 = Concatenate Strings(w215, w216) -> (w217:string)
        n83 = Concatenate Strings(w213, w214) -> (w218:string)
        n84 = call <vilib>:"Build State String with Arguments__JKI_lib_State_Machine.vi"("Arguments (\"\")"=w210, "State"=w212) -> ("State with Arguments"=w209:string)  [unwired: 4 in]
        n85 = call-poly "Build Message with Arguments++.vi"("State With Arguments"="SubMessage1", "Target Module (\"\")"=w199) -> ("CSM Message String"=w204:string)  [unwired: 13 in]
        n86 = call-poly "Build Message with Arguments++.vi"("State With Arguments"="SubMessage2", "Target Module (\"\")"=w199) -> ("CSM Message String"=w203:string)  [unwired: 13 in]
        n87 = call <vilib>:"Build State String with Arguments__JKI_lib_State_Machine.vi"("Arguments (\"\")"=w200, "State"="SubMessage3" ("State With Arguments")) -> ("State with Arguments"=w220:string)  [unwired: 4 in]
        n88 = call-poly "Build Message with Arguments++.vi"("State With Arguments"="Message", "Target Module (\"\")"=w199) -> ("CSM Message String"=w205:string)  [unwired: 13 in]
        n89 = call <vilib>:"Build State String with Arguments__JKI_lib_State_Machine.vi"("Arguments (\"\")"=w217, "State"=w215) -> ("State with Arguments"=w222:string)  [unwired: 4 in]
        n90 = call <vilib>:"Build State String with Arguments__JKI_lib_State_Machine.vi"("Arguments (\"\")"=w218, "State"=w213) -> ("State with Arguments"=w221:string)  [unwired: 4 in]
        n91 = Build Array(w222, w221, w220, w205, w204, w203) -> (w219:string[])
        n92 = call "CSM - Compact Multiple States.vi"("Multiple States"=w219) -> ("States"=w224:string)  [unwired: 9 in]
        n93 = call <vilib>:"Add State(s) to Queue__JKI_lib_State_Machine.vi"("State(s) in Front (\"\")"=w224, "State(s) in (\"\")"=w225, "State(s) at Back (\"\")"=w209) -> ("States Out"=w226:string)  [unwired: 12 in]
      }
      frame "---------- API ----------" {
        # "#CSM \"Category Seperator\"\nDo not put any code in this frame."
      }
      frame "API: Test SyncMessage" {
        n94 = call "CSM - Check If Module Exists.vi"("CSM Name"=w236) -> ("error out"=w230:errorcluster, "Exist?"=w231:bool, "CSM Name (Dup)"=w235:string)  [unwired: 8 in]
        n95 = case shown="True" w231 {
          tunnel: w235 -> [_ w239]
          tunnel: [_ w238] -> w232
          frame False {
          }
          frame True {
            n96 = call "uuid.vi"() -> ("UUID"=w240:string)  [unwired: 11 in]
            n97 = call-poly "Build Message with Arguments++.vi"("State With Arguments"="Message", "Arguments (\"\")"=w240, "Target Module (\"\")"=w239) -> ("CSM Message String"=w238:string)  [unwired: 12 in]
          }
        }
        n98 = call <vilib>:"Add State(s) to Queue__JKI_lib_State_Machine.vi"("State(s) in Front (\"\")"=w232, "State(s) in (\"\")"=w233) -> ("States Out"=w234:string)  [unwired: 13 in]
      }
      frame "API: Test SyncMessage With Error" {
        n99 = call "CSM - Check If Module Exists.vi"("CSM Name"=w248) -> ("error out"=w242:errorcluster, "Exist?"=w243:bool, "CSM Name (Dup)"=w247:string)  [unwired: 8 in]
        n100 = case shown="True" w243 {
          tunnel: w247 -> [_ w251]
          tunnel: [_ w250] -> w244
          frame False {
          }
          frame True {
            n101 = call "uuid.vi"() -> ("UUID"=w252:string)  [unwired: 11 in]
            n102 = call "Build Synchronous Message with Arguments.vi"("State With Arguments"="Message With Error", "Arguments (\"\")"=w252, "Target Module (\"\")"=w251) -> ("CSM Message String"=w250:string)  [unwired: 12 in]
          }
        }
        n103 = call <vilib>:"Add State(s) to Queue__JKI_lib_State_Machine.vi"("State(s) in Front (\"\")"=w244, "State(s) in (\"\")"=w245) -> ("States Out"=w246:string)  [unwired: 13 in]
      }
      frame "API: Test SyncMessage via API" {
        n104 = call "CSM - Check If Module Exists.vi"("CSM Name"=w273) -> ("error out"=w268:errorcluster, "Exist?"=w269:bool, "CSM Name (Dup)"=w272:string)  [unwired: 8 in]
        n105 = case shown="True" w269 {
          tunnel: w272 -> [_ w281]
          tunnel: [_ w280] -> w256
          tunnel: w258 -> [_ w279]
          tunnel: [_ w278] -> w265
          tunnel: [_ w277] -> w255
          tunnel: [_ w276] -> w261
          tunnel: [_ w275] -> w264
          frame False {
          }
          frame True {
            w278 = "Message" ("State With Arguments")
            n106 = call "uuid.vi"() -> ("UUID"=w276:string)  [unwired: 11 in]
            n107 = call "CSM - Wait and Send Message for Reply.vi"("State"=w278, "Current Module (\"\" to Generate an ID)"=w279, "Arguments (\"\")"=w276, "Target Module"=w281) -> ("Response"=w275:string, "Source CSM"=w277:string, "error out"=w280:errorcluster)  [unwired: 8 in, 1 out]
          }
        }
        n108 = call "CSM - Resolve Node Module.vi"("Node Name"=w258) -> ("CSM Module Name"=w257:string)  [unwired: 10 in]
        n109 = call "CSM - Resolve Node Module.vi"("Node Name"=w255) -> ("CSM Module Name"=w254:string)  [unwired: 10 in]
        n110 = Bundle By Name(cluster=T1 {"Arguments"="", "Response"="", "error"={"status"=FALSE, "code"=0, "source"=""}}, "Arguments"=w261, "Response"=w264, "error"=w256) -> (w259:T1)
        n111 = Concatenate Strings(w254, ":" ("string"), w265) -> (w263:string)
        n112 = call "CSM - Set Module Attribute.vi"("CSM Name"=w257, "Attribute"=w263, "Value"=w259) -> ("error out"=w262:errorcluster)  [unwired: 9 in, 3 out]
        n113 = call <vilib>:"Add State(s) to Queue__JKI_lib_State_Machine.vi"("State(s) in (\"\")"=w270) -> ("States Out"=w271:string)  [unwired: 14 in]
        n114 = Merge Errors(w262, w256, w268) -> (w267:errorcluster)
      }
      frame "API: Test SyncMessage With Error via API" {
        n115 = call "CSM - Check If Module Exists.vi"("CSM Name"=w301) -> ("error out"=w296:errorcluster, "Exist?"=w297:bool, "CSM Name (Dup)"=w300:string)  [unwired: 8 in]
        n116 = case shown="True" w297 {
          tunnel: w300 -> [_ w309]
          tunnel: [_ w308] -> w284
          tunnel: w286 -> [_ w307]
          tunnel: [_ w306] -> w293
          tunnel: [_ w305] -> w283
          tunnel: [_ w304] -> w289
          tunnel: [_ w303] -> w292
          frame False {
          }
          frame True {
            w306 = "Message With Error" ("State With Arguments")
            n117 = call "uuid.vi"() -> ("UUID"=w304:string)  [unwired: 11 in]
            n118 = call "CSM - Wait and Send Message for Reply.vi"("State"=w306, "Current Module (\"\" to Generate an ID)"=w307, "Arguments (\"\")"=w304, "Target Module"=w309) -> ("Response"=w303:string, "Source CSM"=w305:string, "error out"=w308:errorcluster)  [unwired: 8 in, 1 out]
          }
        }
        n119 = call "CSM - Resolve Node Module.vi"("Node Name"=w283) -> ("CSM Module Name"=w282:string)  [unwired: 10 in]
        n120 = Bundle By Name(cluster=T1 {"Arguments"="", "Response"="", "error"={"status"=FALSE, "code"=0, "source"=""}}, "Arguments"=w289, "Response"=w292, "error"=w284) -> (w288:T1)
        n121 = call "CSM - Resolve Node Module.vi"("Node Name"=w286) -> ("CSM Module Name"=w285:string)  [unwired: 10 in]
        n122 = Concatenate Strings(w282, ":" ("string"), w293) -> (w291:string)
        n123 = call "CSM - Set Module Attribute.vi"("CSM Name"=w285, "Attribute"=w291, "Value"=w288) -> ("error out"=w290:errorcluster)  [unwired: 9 in, 3 out]
        n124 = call <vilib>:"Add State(s) to Queue__JKI_lib_State_Machine.vi"("State(s) in (\"\")"=w298) -> ("States Out"=w299:string)  [unwired: 14 in]
        n125 = Merge Errors(w290, w284, w296) -> (w295:errorcluster)
      }
      frame "API: Test AsyncMessageWithReply" {
        n126 = call "CSM - Check If Module Exists.vi"("CSM Name"=w316) -> ("error out"=w310:errorcluster, "Exist?"=w311:bool, "CSM Name (Dup)"=w315:string)  [unwired: 8 in]
        n127 = case shown="True" w311 {
          tunnel: w315 -> [_ w319]
          tunnel: [_ w318] -> w312
          frame False {
          }
          frame True {
            n128 = call "uuid.vi"() -> ("UUID"=w320:string)  [unwired: 11 in]
            n129 = call-poly "Build Message with Arguments++.vi"("State With Arguments"="Message", "Arguments (\"\")"=w320, "Target Module (\"\")"=w319) -> ("CSM Message String"=w318:string)  [unwired: 12 in]
          }
        }
        n130 = call <vilib>:"Add State(s) to Queue__JKI_lib_State_Machine.vi"("State(s) in Front (\"\")"=w312, "State(s) in (\"\")"=w313) -> ("States Out"=w314:string)  [unwired: 13 in]
      }
      frame "API: Test AsyncMessageWithReply With Error" {
        n131 = call "CSM - Check If Module Exists.vi"("CSM Name"=w328) -> ("error out"=w322:errorcluster, "Exist?"=w323:bool, "CSM Name (Dup)"=w327:string)  [unwired: 8 in]
        n132 = case shown="True" w323 {
          tunnel: w327 -> [_ w332]
          tunnel: [_ w330] -> w324
          frame False {
          }
          frame True {
            n133 = call "uuid.vi"() -> ("UUID"=w331:string)  [unwired: 11 in]
            n134 = call-poly "Build Message with Arguments++.vi"("State With Arguments"="Message With Error", "Arguments (\"\")"=w331, "Target Module (\"\")"=w332) -> ("CSM Message String"=w330:string)  [unwired: 12 in]
          }
        }
        n135 = call <vilib>:"Add State(s) to Queue__JKI_lib_State_Machine.vi"("State(s) in Front (\"\")"=w324, "State(s) in (\"\")"=w325) -> ("States Out"=w326:string)  [unwired: 13 in]
      }
      frame "API: Test AsyncMessageWithoutReply" {
        n136 = call "CSM - Check If Module Exists.vi"("CSM Name"=w340) -> ("error out"=w334:errorcluster, "Exist?"=w335:bool, "CSM Name (Dup)"=w339:string)  [unwired: 8 in]
        n137 = case shown="True" w335 {
          tunnel: w339 -> [_ w345]
          tunnel: [_ w343] -> w336
          frame False {
          }
          frame True {
            n138 = call-poly "Build Message with Arguments++.vi"("State With Arguments"="AsyncMessageWithoutReply", "Arguments (\"\")"="123456789" ("Arguments (\"\")"), "Target Module (\"\")"=w345) -> ("CSM Message String"=w343:string)  [unwired: 12 in]
          }
        }
        n139 = call <vilib>:"Add State(s) to Queue__JKI_lib_State_Machine.vi"("State(s) in Front (\"\")"=w336, "State(s) in (\"\")"=w337) -> ("States Out"=w338:string)  [unwired: 13 in]
      }
      frame "API: Test AsyncMessageWithoutReply via API" {
        n140 = call "CSM - Check If Module Exists.vi"("CSM Name"=w354) -> ("error out"=w349:errorcluster, "Exist?"=w350:bool, "CSM Name (Dup)"=w353:string)  [unwired: 8 in]
        n141 = case shown="True" w350 {
          tunnel: w353 -> [_ w357]
          tunnel: w348 -> [_ w360]
          tunnel: [_ w356] -> w346
          frame False {
          }
          frame True {
            n142 = call "CSM - Wait and Post Message.vi"("State"="AsyncMessageWithoutReply" ("State With Arguments"), "Current Module (\"\" to Generate an ID)"=w360, "Arguments (\"\")"="123456789" ("Arguments (\"\")"), "Target Module"=w357) -> ("error out"=w356:errorcluster)  [unwired: 10 in, 1 out]
          }
        }
        n143 = call <vilib>:"Add State(s) to Queue__JKI_lib_State_Machine.vi"("State(s) in (\"\")"=w351) -> ("States Out"=w352:string)  [unwired: 14 in]
        n144 = Merge Errors(w346, w349) -> (w347:errorcluster)
      }
      frame "API: Test Argument" {
        n145 = call "uuid.vi"() -> ("UUID"=w366:string)  [unwired: 11 in]
        n146 = call "CSM - Convert HexStr to Data.vi"("HEX String"=w370) -> ("Variant"=w368:variant, "error out"=w369:errorcluster)  [unwired: 7 in]
        n147 = Bundle("", "UUID"=w366) -> (w364:cluster{string, "UUID":string})  [unwired: 1 in]
        n148 = Variant To Data(error in=w369, type=w364, Variant=w368) -> (data=w363:cluster{string, "UUID":string}, error out=w367:errorcluster)
        n149 = Unbundle(w363) -> (w362:string, "UUID"=w361:string)
        n150 = call "CSM - Check If Module Exists.vi"("Error In"=w367, "CSM Name"=w362) -> ("error out"=w371:errorcluster, "Exist?"=w372:bool, "CSM Name (Dup)"=w376:string)  [unwired: 7 in]
        n151 = case shown="True" w372 {
          tunnel: w376 -> [_ w380]
          tunnel: [_ w379] -> w373
          tunnel: w361 -> [_ w378]
          frame False {
          }
          frame True {
            n152 = call "Build Synchronous Message with Arguments.vi"("State With Arguments"="ArgumentTest", "Arguments (\"\")"=w378, "Target Module (\"\")"=w380) -> ("CSM Message String"=w379:string)  [unwired: 12 in]
          }
        }
        n153 = call <vilib>:"Add State(s) to Queue__JKI_lib_State_Machine.vi"("State(s) in Front (\"\")"=w373, "State(s) in (\"\")"=w374) -> ("States Out"=w375:string)  [unwired: 13 in]
      }
      frame "API: Test Response With Error" {
        n154 = call "CSM - Check If Module Exists.vi"("CSM Name"=w388) -> ("error out"=w382:errorcluster, "Exist?"=w383:bool, "CSM Name (Dup)"=w387:string)  [unwired: 8 in]
        n155 = case shown="True" w383 {
          tunnel: w387 -> [_ w391]
          tunnel: [_ w390] -> w384
          frame False {
          }
          frame True {
            n156 = call "uuid.vi"() -> ("UUID"=w392:string)  [unwired: 11 in]
            n157 = call "Build Synchronous Message with Arguments.vi"("State With Arguments"="Response With Error", "Arguments (\"\")"=w392, "Target Module (\"\")"=w391) -> ("CSM Message String"=w390:string)  [unwired: 12 in]
          }
        }
        n158 = call <vilib>:"Add State(s) to Queue__JKI_lib_State_Machine.vi"("State(s) in Front (\"\")"=w384, "State(s) in (\"\")"=w385) -> ("States Out"=w386:string)  [unwired: 13 in]
      }
      frame "API: Test MacroWithSubMessages" {
        n159 = call <vilib>:"Build State String with Arguments__JKI_lib_State_Machine.vi"("Arguments (\"\")"=w395, "State"="Macro: Test MacroWithSubMessages") -> ("State with Arguments"=w394:string)  [unwired: 4 in]
        n160 = call <vilib>:"Add State(s) to Queue__JKI_lib_State_Machine.vi"("State(s) in Front (\"\")"=w394, "State(s) in (\"\")"=w398) -> ("States Out"=w397:string)  [unwired: 13 in]
      }
      frame "API: Test MacroWithSubAndPostMessages" {
        n161 = call <vilib>:"Build State String with Arguments__JKI_lib_State_Machine.vi"("Arguments (\"\")"=w402, "State"="Macro: Test MacroWithSubAndPostMessages") -> ("State with Arguments"=w401:string)  [unwired: 4 in]
        n162 = call <vilib>:"Add State(s) to Queue__JKI_lib_State_Machine.vi"("State(s) in Front (\"\")"=w401, "State(s) in (\"\")"=w405) -> ("States Out"=w404:string)  [unwired: 13 in]
      }
      frame "API: Test MacroWithNonLocalSubMessages" {
        n163 = call <vilib>:"Build State String with Arguments__JKI_lib_State_Machine.vi"("Arguments (\"\")"=w409, "State"="Macro: TestMacroWithNonLocalSubMessages") -> ("State with Arguments"=w408:string)  [unwired: 4 in]
        n164 = call <vilib>:"Add State(s) to Queue__JKI_lib_State_Machine.vi"("State(s) in Front (\"\")"=w408, "State(s) in (\"\")"=w412) -> ("States Out"=w411:string)  [unwired: 13 in]
      }
      frame "API: Test Register State" {
        n165 = call <vilib>:"Build State String with Arguments__JKI_lib_State_Machine.vi"("Arguments (\"\")"=w416, "State"="Test Status") -> ("State with Arguments"=w415:string)  [unwired: 4 in]
        n166 = call <vilib>:"Add State(s) to Queue__JKI_lib_State_Machine.vi"("State(s) in Front (\"\")"=w415, "State(s) in (\"\")"=w419) -> ("States Out"=w418:string)  [unwired: 13 in]
      }
      frame "API: Test Register State Argument Info" {
        n167 = call <vilib>:"Build State String with Arguments__JKI_lib_State_Machine.vi"("Arguments (\"\")"=w423, "State"="Register State Argument Info") -> ("State with Arguments"=w422:string)  [unwired: 4 in]
        n168 = call <vilib>:"Add State(s) to Queue__JKI_lib_State_Machine.vi"("State(s) in Front (\"\")"=w422, "State(s) in (\"\")"=w426) -> ("States Out"=w425:string)  [unwired: 13 in]
      }
      frame "API: Test Register Status" {
        n169 = disable-structure shown="Enabled" {
          disable-tunnel: w431 -> [w441 w442]
          disable-tunnel: [w440 w442] -> w432
          disable-tunnel: w430 -> [w438 _]
          frame Disabled {
            n170 = call <vilib>:"Build State String with Arguments__JKI_lib_State_Machine.vi"("Arguments (\"\")"=w438, "State"="Register Status") -> ("State with Arguments"=w437:string)  [unwired: 4 in]
            n171 = call <vilib>:"Add State(s) to Queue__JKI_lib_State_Machine.vi"("State(s) in Front (\"\")"=w437, "State(s) in (\"\")"=w441) -> ("States Out"=w440:string)  [unwired: 13 in]
          }
          frame Enabled {
          }
        }
        n172 = call <vilib>:"Build State String with Arguments__JKI_lib_State_Machine.vi"("Arguments (\"\")"=w430, "State"="Test Status") -> ("State with Arguments"=w433:string)  [unwired: 4 in]
        n173 = call "CSM - Broadcast Status Change.vi"("Status With Arguments"=w433, "State Queue"=w432) -> ("Remaining States"=w429:string)  [unwired: 13 in]
      }
      frame "API: Test Register Interrupt" {
        n174 = disable-structure shown="Enabled" {
          disable-tunnel: w445 -> [w455 w456]
          disable-tunnel: [w454 w456] -> w446
          disable-tunnel: w444 -> [w452 _]
          frame Disabled {
            n175 = call <vilib>:"Build State String with Arguments__JKI_lib_State_Machine.vi"("Arguments (\"\")"=w452, "State"="Register Interrupt") -> ("State with Arguments"=w451:string)  [unwired: 4 in]
            n176 = call <vilib>:"Add State(s) to Queue__JKI_lib_State_Machine.vi"("State(s) in Front (\"\")"=w451, "State(s) in (\"\")"=w455) -> ("States Out"=w454:string)  [unwired: 13 in]
          }
          frame Enabled {
          }
        }
        n177 = call-poly "Build Message with Arguments++.vi"("State With Arguments"="Test Interrupt", "Arguments (\"\")"=w444) -> ("CSM Message String"=w447:string)  [unwired: 13 in]
        n178 = call <vilib>:"Add State(s) to Queue__JKI_lib_State_Machine.vi"("State(s) in Front (\"\")"=w447, "State(s) in (\"\")"=w446) -> ("States Out"=w443:string)  [unwired: 13 in]
      }
      frame "API: Test Register Status Argument Info" {
        n179 = call <vilib>:"Build State String with Arguments__JKI_lib_State_Machine.vi"("Arguments (\"\")"=w458, "State"="Register Status Argument Info") -> ("State with Arguments"=w457:string)  [unwired: 4 in]
        n180 = call <vilib>:"Add State(s) to Queue__JKI_lib_State_Machine.vi"("State(s) in Front (\"\")"=w457, "State(s) in (\"\")"=w461) -> ("States Out"=w460:string)  [unwired: 13 in]
      }
      frame "API: Test Status A" {
        n181 = call <vilib>:"Build State String with Arguments__JKI_lib_State_Machine.vi"("Arguments (\"\")"=w465, "State"="Broadcast Status A") -> ("State with Arguments"=w466:string)  [unwired: 4 in]
        n182 = call <vilib>:"Add State(s) to Queue__JKI_lib_State_Machine.vi"("State(s) in Front (\"\")"=w466, "State(s) in (\"\")"=w468) -> ("States Out"=w467:string)  [unwired: 13 in]
      }
      frame "API: Test State A" {
        n183 = call <vilib>:"Build State String with Arguments__JKI_lib_State_Machine.vi"("Arguments (\"\")"=w472, "State"="State A") -> ("State with Arguments"=w473:string)  [unwired: 4 in]
        n184 = call <vilib>:"Add State(s) to Queue__JKI_lib_State_Machine.vi"("State(s) in Front (\"\")"=w473, "State(s) in (\"\")"=w475) -> ("States Out"=w474:string)  [unwired: 13 in]
      }
      frame "API: Test State B" {
        n185 = call <vilib>:"Build State String with Arguments__JKI_lib_State_Machine.vi"("Arguments (\"\")"=w479, "State"="State B") -> ("State with Arguments"=w480:string)  [unwired: 4 in]
        n186 = call <vilib>:"Add State(s) to Queue__JKI_lib_State_Machine.vi"("State(s) in Front (\"\")"=w480, "State(s) in (\"\")"=w482) -> ("States Out"=w481:string)  [unwired: 13 in]
      }
      frame "API: Test Status B" {
        n187 = call <vilib>:"Build State String with Arguments__JKI_lib_State_Machine.vi"("Arguments (\"\")"=w486, "State"="Broadcast Status B") -> ("State with Arguments"=w487:string)  [unwired: 4 in]
        n188 = call <vilib>:"Add State(s) to Queue__JKI_lib_State_Machine.vi"("State(s) in Front (\"\")"=w487, "State(s) in (\"\")"=w489) -> ("States Out"=w488:string)  [unwired: 13 in]
      }
      frame "API: Local Registration" {
        # "Test Status @ From >> Handler Message @ To -><register>"
        n189 = call "CSM - Resolve Node Module.vi"("Node Name"=w496) -> ("CSM Module Name"=w492:string)  [unwired: 10 in]
        n190 = call-poly "Build Message with Arguments++.vi"("Target CSM"=w493, "Source CSM (* as Default)"=w492, "Status"="Test Status", "API (If \"\", Same As \"Status\")"="Handler Message") -> ("CSM Message String"=w494:string)  [unwired: 11 in]
        n191 = call <vilib>:"Add State(s) to Queue__JKI_lib_State_Machine.vi"("State(s) in Front (\"\")"=w494, "State(s) in (\"\")"=w500) -> ("States Out"=w499:string)  [unwired: 13 in]
      }
      frame "API: Local Registration II" {
        # "Test Status @ From >> Handler Message -><register>"
        n192 = call "CSM - Resolve Node Module.vi"("Node Name"=w504) -> ("CSM Module Name"=w501:string)  [unwired: 10 in]
        n193 = call-poly "Build Message with Arguments++.vi"("Source CSM (* as Default)"=w501, "Status"="Test Status", "API (If \"\", Same As \"Status\")"="Handler Message") -> ("CSM Message String"=w502:string)  [unwired: 12 in]
        n194 = call <vilib>:"Add State(s) to Queue__JKI_lib_State_Machine.vi"("State(s) in Front (\"\")"=w502, "State(s) in (\"\")"=w508) -> ("States Out"=w507:string)  [unwired: 13 in]
      }
      frame "API: Local Unregistration" {
        # "Test Status @ From >> Handler Message @ To -><unregister>"
        n195 = call "CSM - Resolve Node Module.vi"("Node Name"=w513) -> ("CSM Module Name"=w509:string)  [unwired: 10 in]
        n196 = call-poly "Build Message with Arguments++.vi"("Target CSM"=w510, "Source CSM (* as Default)"=w509, "Status"="Test Status", "API (If \"\", Same As \"Status\")"="Handler Message") -> ("CSM Message String"=w511:string)  [unwired: 11 in]
        n197 = call <vilib>:"Add State(s) to Queue__JKI_lib_State_Machine.vi"("State(s) in Front (\"\")"=w511, "State(s) in (\"\")"=w517) -> ("States Out"=w516:string)  [unwired: 13 in]
      }
      frame "API: Local Registration via API" {
        # "Test Status @ From >> Handler Message @ To -><register>"
        n198 = call "CSM - Resolve Node Module.vi"("Node Name"=w523) -> ("CSM Module Name"=w519:string)  [unwired: 10 in]
        n199 = call "CSM - Register Broadcast.vi"("CSM Name(Empty for Broadcast Event)"=w518, "Source CSM Name (* as Default)"=w519, "Trigger"="Test Status", "API (If \"\", Same as Trigger)"="Handler Message") -> ("error out"=w522:errorcluster)  [unwired: 10 in, 1 out]
        n200 = call <vilib>:"Add State(s) to Queue__JKI_lib_State_Machine.vi"("State(s) in (\"\")"=w526) -> ("States Out"=w525:string)  [unwired: 14 in]
      }
      frame "API: Local Unregistration via API" {
        # "Test Status @ From >> Handler Message @ To -><unregister>"
        n201 = call "CSM - Resolve Node Module.vi"("Node Name"=w532) -> ("CSM Module Name"=w528:string)  [unwired: 10 in]
        n202 = call "CSM - Unregister Broadcast.vi"("CSM Name(Empty for Broadcast Event)"=w527, "Source CSM Name (* as Default)"=w528, "Trigger"="Test Status", "API (\"*\" as Default)"="Handler Message") -> ("error out"=w531:errorcluster)  [unwired: 10 in, 1 out]
        n203 = call <vilib>:"Add State(s) to Queue__JKI_lib_State_Machine.vi"("State(s) in (\"\")"=w535) -> ("States Out"=w534:string)  [unwired: 14 in]
      }
      frame "API: Start CSM Loop" {
        n204 = call <vilib>:"Add State(s) to Queue__JKI_lib_State_Machine.vi"("State(s) in Front (\"\")"="Macro: Start CSM Loop" ("State(s) in Front (\"\")"), "State(s) in (\"\")"=w538) -> ("States Out"=w537:string)  [unwired: 13 in]
      }
      frame "API: Stop CSM Loop" {
        n205 = call <vilib>:"Add State(s) to Queue__JKI_lib_State_Machine.vi"("State(s) in Front (\"\")"="Macro: Stop CSM Loop" ("State(s) in Front (\"\")"), "State(s) in (\"\")"=w542) -> ("States Out"=w541:string)  [unwired: 13 in]
      }
      frame "API: API2" {
        # "#CSM API Example\nCopy/Rename this case for your own API"
        # "unpack Hex String  to Variant\nif complex parameter is needed."
        n206 = call "CSM - Convert HexStr to Data.vi"("HEX String"=w547) -> ()  [unwired: 7 in, 2 out]
        n207 = disable-structure shown="Enabled" {
          disable-tunnel: [w550 "API2 Response"] -> w546
          frame Disabled {
            # "pack variant to hexstr \nif complex response is needed."
            # "complex Response"
            n208 = call "CSM - Convert Data to HexStr.vi"() -> ("HEX String (0-9,A-F)"=w550:string)  [unwired: 9 in]
          }
          frame Enabled {
          }
        }
      }
      frame "---------- Action ----------" {
        # "#CSM \"Category Seperator\"\nDo not put any code in this frame."
        n209 = call <vilib>:"Add State(s) to Queue__JKI_lib_State_Machine.vi"("State(s) in (\"\")"=w554) -> ("States Out"=w553:string)  [unwired: 14 in]
      }
      frame "Action: action1" {
        # "#CSM \"Internal State\"\nThis category is used for holding internal states"
        n210 = call <vilib>:"Add State(s) to Queue__JKI_lib_State_Machine.vi"("State(s) in (\"\")"=w557) -> ("States Out"=w556:string)  [unwired: 14 in]
      }
      frame "Start CSM Loop" {
        n211 = Bundle By Name(cluster=w560, "CSM Loop Counter"=0) -> (w559:T6)
      }
      frame "Run CSM Loop" {
        n212 = Wait (ms)(milliseconds to wait=u32 50) -> ()  [unwired: 1 out]
        n213 = Unbundle By Name(w571) -> ("CSM Loop Counter"=w570:i32)
        n214 = call "CSM - Resolve Node Module.vi"("Node Name"=w567) -> ("CSM Module Name"=w566:string)  [unwired: 10 in]
        n215 = Increment(x=w570) -> (x+1=w564:i32)
        n216 = Bundle By Name(cluster=w571, "CSM Loop Counter"=w564) -> (w569:T6)
        n217 = call "CSM - Set Module Attribute.vi"("CSM Name"=w566, "Attribute"=w565, "Value"=w564) -> ("error out"=w563:errorcluster)  [unwired: 9 in, 3 out]
        n218 = call "CSMLS - Append Continuous State.vi"("Append? (T)"=TRUE, "Continous State"=w565, "States Queue"=w573) -> ("Remaining States"=w574:string)  [unwired: 8 in]
      }
      frame "Stop CSM Loop" {
        w576 = -1 ("CSM Loop Counter")
        n219 = call "CSM - Resolve Node Module.vi"("Node Name"=w577) -> ("CSM Module Name"=w579:string)  [unwired: 10 in]
        n220 = Bundle By Name(cluster=w581, "CSM Loop Counter"=w576) -> (w580:T6)
        n221 = call "CSM - Set Module Attribute.vi"("CSM Name"=w579, "Attribute"=w575, "Value"=w576) -> ("error out"=w578:errorcluster)  [unwired: 9 in, 3 out]
        n222 = call "CSMLS - Remove Loop Tag and previous State(s) to Break.vi"("States Queue"=w583) -> ("Remaining States"=w582:string)  [unwired: 10 in]
        n223 = call <vilib>:"Add State(s) to Queue__JKI_lib_State_Machine.vi"("State(s) in (\"\")"=w582) -> ("States Out"=w584:string)  [unwired: 14 in]
      }
      frame "Test Status" {
        n224 = call <vilib>:"Add State(s) to Queue__JKI_lib_State_Machine.vi"("State(s) in (\"\")"=w588) -> ("States Out"=w587:string)  [unwired: 14 in]
      }
      frame "Register State Argument Info" {
        n225 = call "CSM - Resolve Node Module.vi"("Node Name"=w591) -> ("CSM Module Name"=w592:string)  [unwired: 10 in]
        n226 = Concatenate Strings(w589, "+", w592) -> (w590:string)
        n227 = call <vilib>:"Add State(s) to Queue__JKI_lib_State_Machine.vi"("State(s) in (\"\")"=w594) -> ("States Out"=w596:string)  [unwired: 14 in]
      }
      frame "Register Status" {
        n228 = call <vilib>:"Build State String with Arguments__JKI_lib_State_Machine.vi"("Arguments (\"\")"=w597, "State"="Test Status") -> ("State with Arguments"=w599:string)  [unwired: 4 in]
        n229 = call "CSM - Broadcast Status Change.vi"("Status With Arguments"=w599, "State Queue"=w601) -> ("Remaining States"=w598:string)  [unwired: 13 in]
      }
      frame "Register Interrupt" {
        n230 = call-poly "Build Message with Arguments++.vi"("State With Arguments"="Test Interrupt", "Arguments (\"\")"=w606) -> ("CSM Message String"=w605:string)  [unwired: 13 in]
        n231 = call <vilib>:"Add State(s) to Queue__JKI_lib_State_Machine.vi"("State(s) in Front (\"\")"=w605, "State(s) in (\"\")"=w604) -> ("States Out"=w603:string)  [unwired: 13 in]
      }
      frame "Register Status Argument Info" {
        w613 = "Test Status Argument Info"
        n232 = call "CSM - Resolve Node Module.vi"("Node Name"=w611) -> ("CSM Module Name"=w610:string)  [unwired: 10 in]
        n233 = Concatenate Strings(w613, "+", w610) -> (w609:string)
        n234 = call <vilib>:"Build State String with Arguments__JKI_lib_State_Machine.vi"("Arguments (\"\")"=w609, "State"=w613) -> ("State with Arguments"=w615:string)  [unwired: 4 in]
        n235 = call "CSM - Broadcast Status Change.vi"("Status With Arguments"=w615, "State Queue"=w616) -> ("Remaining States"=w614:string)  [unwired: 13 in]
      }
      frame "Broadcast Status A" {
        n236 = call <vilib>:"Build State String with Arguments__JKI_lib_State_Machine.vi"("Arguments (\"\")"=w618, "State"="Status A") -> ("State with Arguments"=w620:string)  [unwired: 4 in]
        n237 = call "CSM - Broadcast Status Change.vi"("Status With Arguments"=w620, "State Queue"=w622) -> ("Remaining States"=w619:string)  [unwired: 13 in]
      }
      frame "Broadcast Status B" {
        n238 = call <vilib>:"Build State String with Arguments__JKI_lib_State_Machine.vi"("Arguments (\"\")"=w624, "State"="Status B") -> ("State with Arguments"=w626:string)  [unwired: 4 in]
        n239 = call "CSM - Broadcast Status Change.vi"("Status With Arguments"=w626, "State Queue"=w628) -> ("Remaining States"=w625:string)  [unwired: 13 in]
      }
      frame "State A" {
        n240 = call <vilib>:"Add State(s) to Queue__JKI_lib_State_Machine.vi"("State(s) in (\"\")"=w632) -> ("States Out"=w631:string)  [unwired: 14 in]
      }
      frame "State B" {
        n241 = call <vilib>:"Add State(s) to Queue__JKI_lib_State_Machine.vi"("State(s) in (\"\")"=w637) -> ("States Out"=w636:string)  [unwired: 14 in]
      }
      frame "Message" {
      }
      frame "SubMessage1" {
      }
      frame "SubMessage2" {
      }
      frame "SubMessage3" {
        n242 = call "CSM - Resolve Node Module.vi"("Node Name"=w657) -> ("CSM Module Name"=w656:string)  [unwired: 10 in]
        n243 = call "CSM - Set Module Attribute.vi"("CSM Name"=w656, "Attribute"=w655, "Value"=w654) -> ("error out"=w652:errorcluster)  [unwired: 9 in, 3 out]
        n244 = Merge Errors(w652, w660) -> (w653:errorcluster)
      }
      frame "PostMessage1" {
      }
      frame "Message With Error" {
        n245 = Merge Errors(errorcluster {"status"=TRUE, "code"=1234567898, "source"="Simulated Error\nwill be sent to Response case"} ("error out"), w666) -> (w665:errorcluster)
      }
      frame "Response With Error" {
        n246 = Merge Errors(errorcluster {"status"=TRUE, "code"=1234567898, "source"="Simulated Error"} ("error out"), w672) -> (w671:errorcluster)
      }
      frame "ArgumentTest" {
        n247 = call "CSM - Resolve Node Module.vi"("Node Name"=w682) -> ("CSM Module Name"=w681:string)  [unwired: 10 in]
        n248 = call "CSM - Set Module Attribute.vi"("CSM Name"=w681, "Attribute"=w679, "Value"=w680) -> ("error out"=w677:errorcluster)  [unwired: 9 in, 3 out]
        n249 = Merge Errors(w677, w685) -> (w678:errorcluster)
      }
      frame "AsyncMessageWithoutReply" {
        # "123456789 string constant"
        n250 = call "CSM - Resolve Node Module.vi"("Node Name"=w689) -> ("CSM Module Name"=w688:string)  [unwired: 10 in]
        n251 = call "CSM - Set Module Attribute.vi"("CSM Name"=w688, "Attribute"=w690, "Value"=w691) -> ("error out"=w686:errorcluster)  [unwired: 9 in, 3 out]
        n252 = Merge Errors(w686, w694) -> (w687:errorcluster)
      }
      frame "Handler Message" {
        n253 = call "CSM - Resolve Node Module.vi"("Node Name"=w700) -> ("CSM Module Name"=w699:string)  [unwired: 10 in]
        n254 = call "CSM - Set Module Attribute.vi"("CSM Name"=w699, "Attribute"=w697, "Value"=w696) -> ("error out"=w695:errorcluster)  [unwired: 9 in, 3 out]
        n255 = Merge Errors(w703, w695) -> (w698:errorcluster)
      }
      frame "Handler Message With Counter" {
        n256 = Unbundle By Name(w709) -> ("Counter"=w710:u32)
        n257 = Decimal String To Number(string=w707) -> (number=w704:i32)  [unwired: 2 in, 1 out]
        n258 = Increment(x=w710) -> (x+1=w705:u32)
        n259 = Bundle By Name(cluster=w709, "Counter"=w705) -> (w708:T6)
        n260 = Equal?(x=w705, y=w704) -> (x = y?=w706:bool)
        n261 = call "CSM - Resolve Node Module.vi"("Node Name"=w715) -> ("CSM Module Name"=w714:string)  [unwired: 10 in]
        n262 = case shown="True" w706 {
          tunnel: w714 -> [_ w721]
          tunnel: w712 -> [_ w720]
          tunnel: [_ w719] -> w711
          tunnel: w705 -> [_ w718]
          frame False {
          }
          frame True {
            n263 = call "CSM - Set Module Attribute.vi"("CSM Name"=w721, "Attribute"=w720, "Value"=w718) -> ("error out"=w719:errorcluster)  [unwired: 9 in, 3 out]
          }
        }
        n264 = Merge Errors(w717, w711) -> (w713:errorcluster)
      }
      frame "Reset Counter" {
        # "#CSM \"Internal State\"\nThis category is used for holding internal states"
        n265 = Bundle By Name(cluster=w724, "Counter"=u32 0) -> (w722:T6)
        n266 = call <vilib>:"Add State(s) to Queue__JKI_lib_State_Machine.vi"("State(s) in (\"\")"=w726) -> ("States Out"=w725:string)  [unwired: 14 in]
      }
    }
  }
